vi "Connect.vi"(8 "error in (no error)":errorcluster, 11 "NI Vision Camera in":refnum<class "NI Vision Camera.lvclass">) -> (0 "error out":errorcluster, 3 "NI Vision Camera out":refnum<class "NI Vision Camera.lvclass">)   [LabVIEW 2014, in "NI Vision Camera.lvclass"]
uses:
  NI Vision Camera.lvclass
  NI Vision Camera Device/NI Vision Camera Device.lvclass
  NI Vision Camera.lvclass/NI Vision Camera.ctl
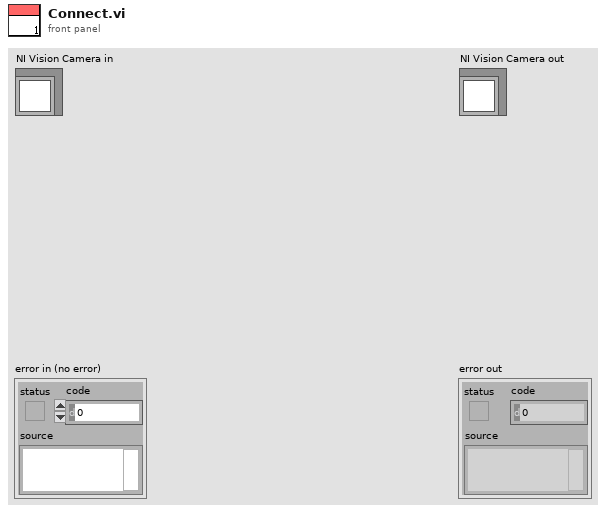
[diagram p1: front panel]
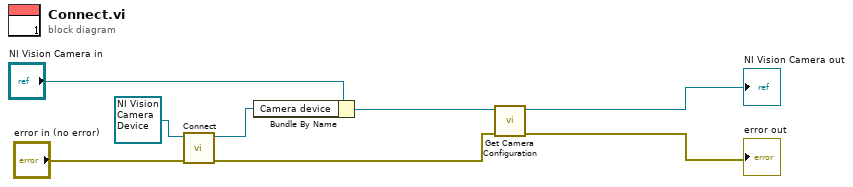
[diagram p0: block diagram]
diagram:
  n1 = call-dynamic "Connect.vi"("error in (no error)"="error in (no error)", "NI Vision Camera Device in"=refnum<class "NI Vision Camera Device.lvclass"> refnum) -> ("error out"=w2:errorcluster, "NI Vision Camera Device out"=w4:refnum<class "NI Vision Camera Device.lvclass">)  [unwired: 8 in]
  n2 = Bundle By Name(cluster="NI Vision Camera in", "Camera device"=w4) -> (w3:refnum<class "NI Vision Camera.lvclass">)
  n3 = call "Get Camera Configuration.vi"("error in (no error)"=w2, "NI Vision Camera in"=w3) -> ("error out"=→"error out":errorcluster, "NI Vision Camera out"=→"NI Vision Camera out":refnum<class "NI Vision Camera.lvclass">)  [unwired: 7 in, 1 out]
